vi "GetUDL_FilePath.vi"() -> (3 "UDL file path":path)   [LabVIEW 2015, in "DatabaseApi.lvlib"]
doc: "This VI is used as a subVI in all the Database Tools example VIs. This VI looks for a file in the Examples/database directory called LabVIEW.udl and returns the path. \n\nA UDL (Universal Data Link) file specifies the connection to an OLE DB provider and a data source. The LabVIEW.udl supplied with the Database Tools examples specifies the Microsoft Jet 4.0 OLE DB Provider connected to the database file named LabVIEW.mdb."
uses:
  DatabaseApi.lvlib
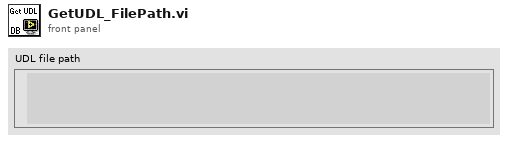
[diagram p1: front panel]
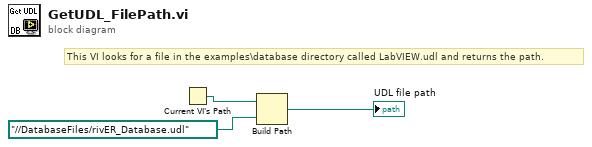
[diagram p0: block diagram]
diagram:
  # "This VI looks for a file in the examples\\database directory called LabVIEW.udl and returns the path."
  n1 = Current VI's Path() -> (path=w1:path)
  n2 = Build Path(base path=w1, name or relative path=path "../../DatabaseFiles/rivER_Database.udl" ("Application:Directory Path")) -> (appended path=→"UDL file path":path)
